vi "Initialize.vi"(8 "error in (no error)":errorcluster, 11 "Stage_MadCityLabMicro in":refnum<class "Stage_MadCityLabMicro.lvclass">) -> (0 "error out":errorcluster, 3 "Stage_MadCityLabMicro out":refnum<class "Stage_MadCityLabMicro.lvclass">)   [LabVIEW 2020, in "Stage_MadCityLabMicro.lvlib" / "Stage_MadCityLabMicro.lvclass"]
uses:
  Stage_MadCityLabMicro.lvclass
  Stage_MadCityLabMicro.lvclass/Stage_MadCityLabMicro.ctl
  HAL Layer/Component/Stage/Stage/Stage.lvclass
  Dependency/MicroDrive.dll
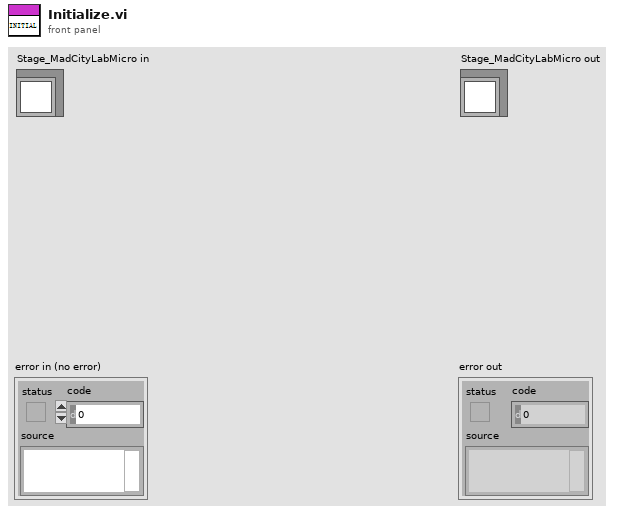
[diagram p1: front panel]
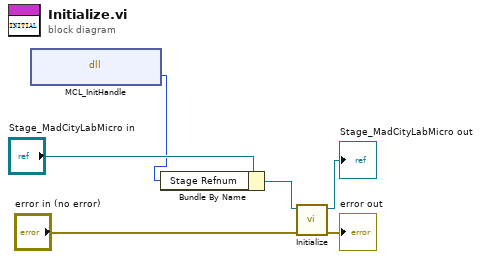
[diagram p0: block diagram]
diagram:
  n1 = dll-call lib="E:/Development/DevHardSoftware/MMicroscopyAF/Model/Real Hardware/Stage_MadCityLabMicro/Stage_MadCityLabMicro/Dependency/MicroDrive.dll" fn="MCL_InitHandle"() -> ("return type"=w1:i32)  [unwired: 3 in, 2 out]
  n2 = Bundle By Name(cluster="Stage_MadCityLabMicro in", "Stage Refnum"=w1) -> (w2:refnum<class "Stage_MadCityLabMicro.lvclass">)
  n3 = call-parent "Initialize.vi"("error in (no error)"="error in (no error)", "Device in"=w2) -> ("error out"=→"error out":errorcluster, "Device out"=→"Stage_MadCityLabMicro out":refnum<class "Stage_MadCityLabMicro.lvclass">)  [unwired: 8 in]
